vi "Launch Calibration.vi"(8 "error in (no error)":errorcluster, 11 "Controller in":refnum<class "Controller.lvclass">) -> (0 "error out":errorcluster, 3 "Controller out":refnum<class "Controller.lvclass">)   [LabVIEW 2022 SP3, in "Controller.lvlib" / "Controller.lvclass"]
uses:
  Controller.lvclass
  Controller.lvclass/Controller.ctl
  <vilib>/ActorFramework/Message Enqueuer/Message Enqueuer.lvclass/Message Enqueuer.ctl
  <vilib>/ActorFramework/Message Enqueuer/Enqueue.vi
  ImageHandler/ImageHandler Messages/DeInit Msg/DeInit Msg.lvclass
  C:/Program Files/National Instruments/LabVIEW 2022/vi.lib/ActorFramework/Message/Message.lvclass
  ImageHandler/ImageHandler Messages/Init Msg/Init Msg.lvclass
  <vilib>/ActorFramework/Message Priority Queue/Priority Enqueue.vi
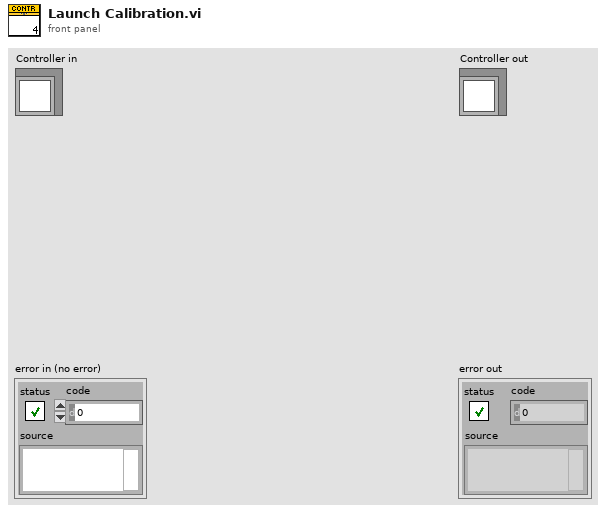
[diagram p1: front panel]
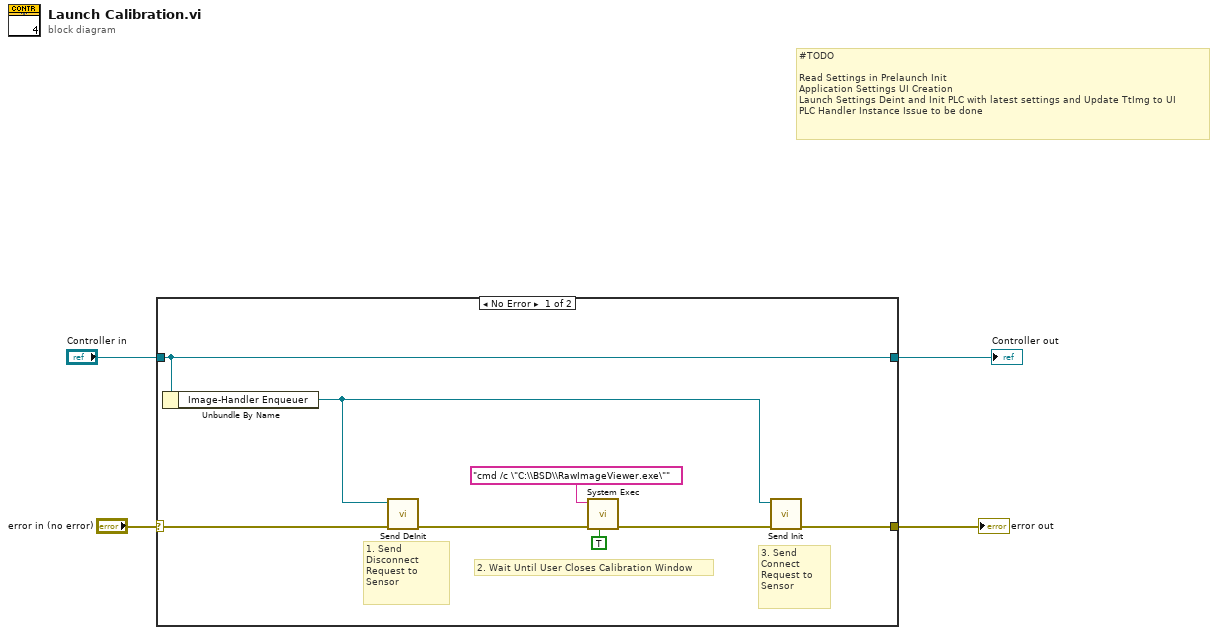
[diagram p0: block diagram]
diagram:
  # "#TODO\n\nRead Settings in Prelaunch Init\nApplication Settings UI Creation\nLaunch Settings Deint and Init PLC with latest settings and Update TtImg to UI\nPLC Handler Instance Issue to be done"
  n1 = case shown="No Error" "error in (no error)" {
    selector: "error in (no error)" -> [w10 w13]
    tunnel: "Controller in" -> [w6 w14]
    tunnel: [w6 w14] -> w2
    tunnel: [w7 w13] -> w1
    frame No Error {
      # "2. Wait Until User Closes Calibration Window"
      # "3. Send Connect Request to Sensor"
      # "1. Send Disconnect Request to Sensor"
      n2 = Unbundle By Name(w6) -> ("Image-Handler Enqueuer"=w5:refnum<class "Message Enqueuer.lvclass">)
      n3 = call "Send DeInit.vi"("error in (no error)"=w10, "Message Enqueuer"=w5) -> ("error out"=w9:errorcluster)  [unwired: 8 in, 1 out]
      n4 = call <vilib>:"System Exec.vi"("run minimized? (F)"=TRUE, "error in (no error)"=w9, "command line"="cmd /c \"C:\\BSD\\RawImageViewer.exe\"") -> ("error out"=w8:errorcluster)  [unwired: 5 in, 3 out]
      n5 = call "Send Init.vi"("error in (no error)"=w8, "Message Enqueuer"=w5) -> ("error out"=w7:errorcluster)  [unwired: 8 in, 1 out]
    }
    frame Error {
    }
  }
  "error out" <- w1
  "Controller out" <- w2
